vi "Initialize.vi"(8 "error in":errorcluster, 10 "parameters":variant, 11 "Thermo Channel in":refnum<class "Thermo Channel.lvclass">) -> (0 "error out":errorcluster, 2 "summary":T2[](array[typedef]), 3 "data value reference":T1)   [LabVIEW 2025, in "Thermo.lvlib" / "Thermo Channel.lvclass"]
doc: "This Vi initializes the data of a node its default state.\nThe object is not created inside of this ViI, beacuase it is created from a File depending on user selection.Copyright 2017 National Instruments Corporation\n\nLicensed under the Apache License, Version 2.0 (the \"License\"); you may not use this file except in compliance with the License. You may obtain a copy of the License at http://www.apache.org/licenses/LICENSE-2.0\nUnless required by applicable law or agreed to in writing, software distributed under the License is distributed on an \"AS IS\" BASIS, WITHOUT WARRANTIES OR CONDITIONS OF ANY KIND, either express or implied. See the License for the specific language governing permissions and limitations under the License."
uses:
  Thermo Channel.lvclass
  Thermo Channel.lvclass/Thermo Channel.ctl
  Users/Public/Documents/Sandia National Labs/TSS Plugin/CEF.lvlibp/Node/CEF_Node.lvclass
  Thermo Instrument/Thermo Instrument.lvclass
  Thermo configuration/Thermo configuration.lvclass
  Users/Public/Documents/Sandia National Labs/TSS Plugin/Abstract Engine.lvlibp/Abstract Channel/Abstract Channel.lvclass
  Thermo Channel configuration/Thermo Channel configuration.lvclass
  Users/Public/Documents/Sandia National Labs/TSS Plugin/CEF.lvlibp/Node/NodeRef.ctl
  Users/Public/Documents/Sandia National Labs/TSS Plugin/CEF.lvlibp/Node/Summary.ctl
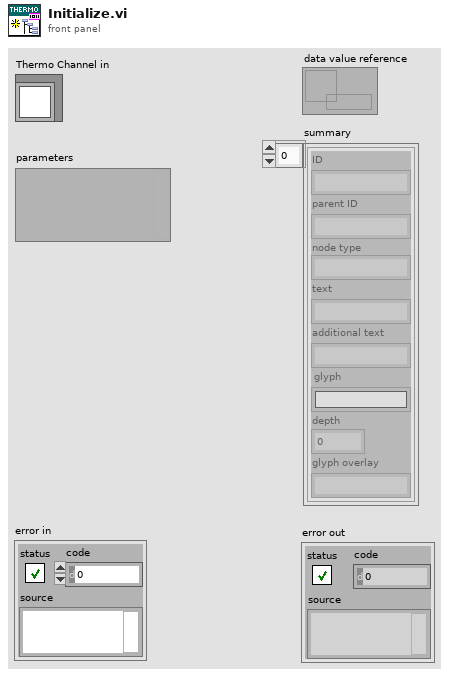
[diagram p1: front panel]
types:
  T1 = typedef "CEF.lvlibp/CEF_Node.lvclass/NodeRef.ctl" = refnum<data-value>
  T2 = typedef "CEF.lvlibp/CEF_Node.lvclass/Summary.ctl" = cluster{"ID":string, "parent ID":string, "node type":string, "text":string, "additional text":string, "glyph":string, "depth":i32, "glyph overlay":string}
  T3 = typedef "Abstract Engine.lvlibp/Instrument configuration.lvclass/Default Instrument.ctl" = cluster{"Type":string, "Address":string, "SW Alias":string, "Description":string, "Enabled":bool}
  T4 = typedef "Abstract Engine.lvlibp/Channel configuration.lvclass/Default Channel.ctl" = cluster{"Address":string, "SW Alias":string, "Enabled":bool, "Type":string, "Description":string}
  T5 = cluster{"ID":string, "parent ID":string, "node type":string, "text":string, "additional text":string, "glyph":string, "depth":i32, "glyph overlay":string}[]
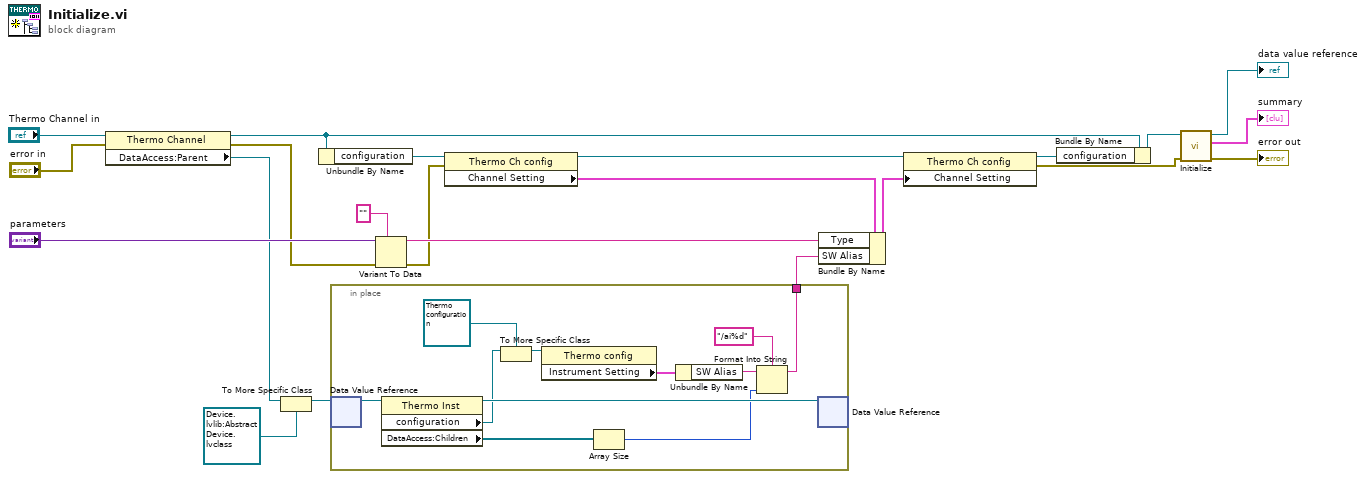
[diagram p0: block diagram]
diagram:
  n1 = property class="Thermo Channel"(reference="Thermo Channel in", error in="error in") -> (reference out=w14:refnum<class "Thermo Channel.lvclass">, error out=w9:errorcluster, "DataAccess:Parent"=w16:refnum<data-value>)
  n2 = To More Specific Class(target class=refnum<data-value> refnum ("data value reference"), reference=w16) -> (specific class reference=w17:refnum<data-value>)  [unwired: 1 in, 1 out]
  n3 = Unbundle By Name(w14) -> ("configuration"=w15:refnum<class "Thermo Channel configuration.lvclass">)
  n4 = in-place {
    in-place-border: [w30] -> w10
    n5 = in-place-dvr #1(w17) -> (w29:refnum<class "Thermo Instrument.lvclass">)  [unwired: 1 out]
    n6 = property class="Thermo Inst"(reference=w29) -> (reference out=w28:refnum<class "Thermo Instrument.lvclass">, "configuration"=w27:refnum<class "CEF_serializable configuration.lvclass">, "DataAccess:Children"=w26:refnum<data-value>[])  [unwired: 1 in, 1 out]
    n7 = To More Specific Class(target class=refnum<class "Thermo configuration.lvclass"> refnum ("Device.lvlib:Device configuration.lvclass"), reference=w27) -> (specific class reference=w33:refnum<class "Thermo configuration.lvclass">)  [unwired: 1 in, 1 out]
    n8 = property class="Thermo config"(reference=w33) -> ("Instrument Setting"=w23:T3)  [unwired: 1 in, 2 out]
    n9 = Array Size(array=w26) -> (size(s)=w25:i32)
    n10 = Unbundle By Name(w23) -> ("SW Alias"=w32:string)
    n11 = Format Into String(format string="/ai%d", initial string=w32, w25) -> (resulting string=w30:string)  [unwired: 1 in, 1 out]
    n12 = in-place-dvr #1(w28) -> ()  [unwired: 2 out]
  }
  n13 = Variant To Data(error in=w9, type="", Variant="parameters") -> (data=w6:string, error out=w5:errorcluster)
  n14 = property class="Thermo Ch config"(reference=w15, error in=w5) -> (reference out=w4:refnum<class "Thermo Channel configuration.lvclass">, "Channel Setting"=w3:T4)  [unwired: 1 out]
  n15 = Bundle By Name(cluster=w3, "Type"=w6, "SW Alias"=w10) -> (w2:T4)
  n16 = property class="Thermo Ch config"(reference=w4, "Channel Setting"=w2) -> (reference out=w12:refnum<class "Thermo Channel configuration.lvclass">, error out=w8:errorcluster)  [unwired: 1 in]
  n17 = Bundle By Name(cluster=w14, "configuration"=w12) -> (w13:refnum<class "Thermo Channel.lvclass">)
  n18 = call-parent "Initialize.vi"("error in"=w8, "CEF_Serialize node in"=w13) -> ("error out"=→"error out":errorcluster, "summary"=→"summary":T5, "data value reference"=→"data value reference":refnum<data-value>)  [unwired: 7 in]
